vi "read_previous_item.vi"(8 "error in (no error)":errorcluster, 9 "Wrap? (F)":bool, 11 "StringList in":refnum<class "StringList.lvclass">) -> (0 "error out":errorcluster, 1 "At Top?":bool, 2 "List Item":string, 3 "StringList out":refnum<class "StringList.lvclass">)   [LabVIEW 2015, in "StringList.lvlib" / "StringList.lvclass"]
uses:
  StringList.lvclass
  StringList.lvclass/StringList.ctl
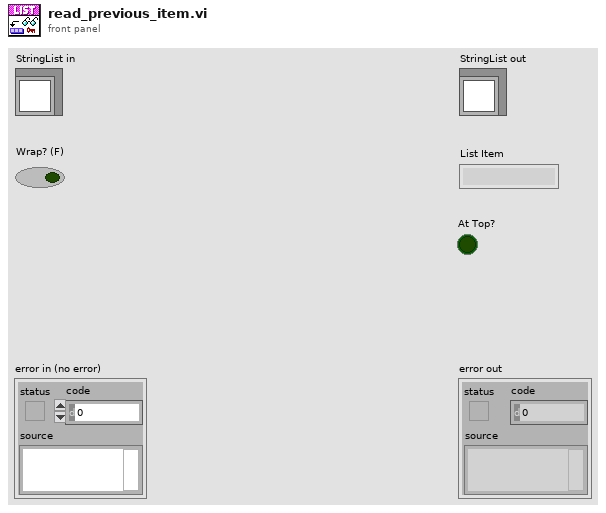
[diagram p1: front panel]
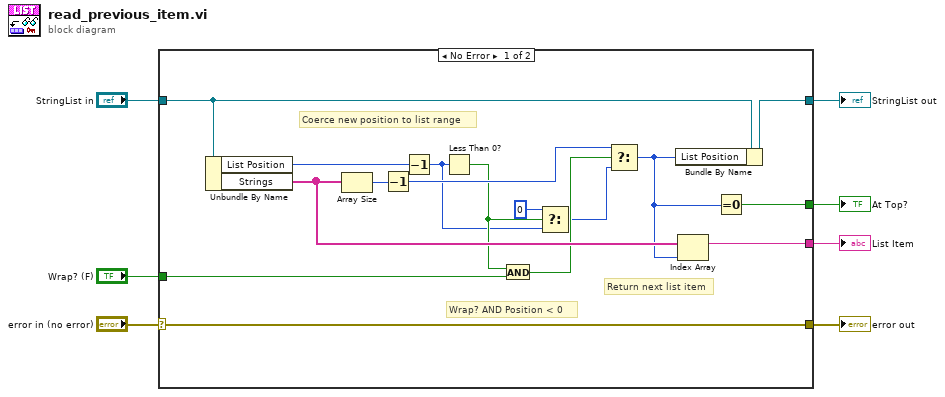
[diagram p0: block diagram]
diagram:
  n1 = case shown="No Error" "error in (no error)" {
    selector: "error in (no error)" -> [w23 w25]
    tunnel: [w23 w25] -> w6
    tunnel: [w20 w24] -> w4
    tunnel: "StringList in" -> [w22 w24]
    tunnel: [w21 _] -> w3
    tunnel: "Wrap? (F)" -> [w10 _]
    tunnel: [w8 _] -> w1
    frame No Error {
      # "Wrap? AND Position < 0"
      # "Coerce new position to list range"
      # "Return next list item"
      n2 = Unbundle By Name(w22) -> ("List Position"=w19:i32, "Strings"=w18:string[])
      n3 = Array Size(array=w18) -> (size(s)=w17:i32)
      n4 = Decrement(x=w17) -> (x-1=w15:i32)
      n5 = Decrement(x=w19) -> (x-1=w12:i32)
      n6 = Less Than 0?(x=w12) -> (x < 0?=w14:bool)
      n7 = And(x=w14, y=w10) -> (x .and. y?=w16:bool)
      n8 = Select(t=0 ("lower limit"), s=w14, f=w12) -> (s? t:f=w11:i32)
      n9 = Select(t=w15, s=w16, f=w11) -> (s? t:f=w9:i32)
      n10 = Bundle By Name(cluster=w22, "List Position"=w9) -> (w20:refnum<class "StringList.lvclass">)
      n11 = Index Array(array=w18, index=w9) -> (element=w21:string)
      n12 = Equal To 0?(x=w9) -> (x = 0?=w8:bool)
    }
    frame Error {
    }
  }
  "error out" <- w6
  "StringList out" <- w4
  "List Item" <- w3
  "At Top?" <- w1
